vi "Tool Q LEIN High G Get buffer size.vi"(11 "error in (no error)":errorcluster) -> (15 "error out":errorcluster)   [LabVIEW 2011]
uses:
  LEINmaster/Defenitions/LEIN Structure variations.ctl
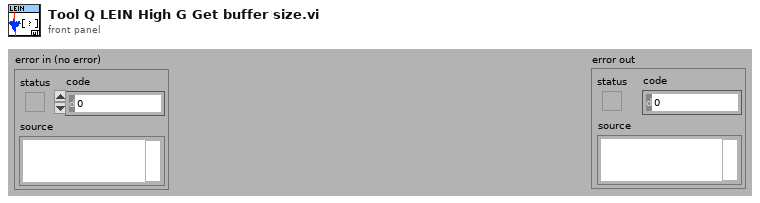
[diagram p1: front panel]
types:
  T1 = typedef "LEIN Structure variations.ctl" = enum16{"LEIN08", "LEIN31", "LEIN63"}
  T2 = typedef "LEIN CMD Cluster.ctl" = cluster{"SID":u8, "ANF":bool, "CMD":T3, "DATA":u8[]}
  T3 = typedef "LEIN CMD List.ctl" = enum8{"ACTI", "TASK", "RES0", "STAT", "RES1", "RES2", "RES3", "USER"}
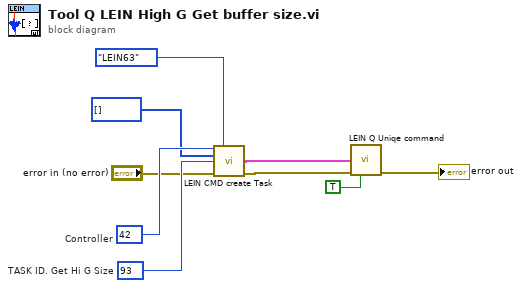
[diagram p0: block diagram]
diagram:
  w5 = u8 42  # Controller
  w7 = u8 93  # TASK ID. Get Hi G Size
  n1 = call "LEIN CMD create Task.vi"("SID"=w5, "LEIN Variation"=LEIN_Structure_variations."LEIN63", "Data"=u8[] [], "TASK ID"=w7, "error in (no error)"="error in (no error)") -> ("CMD"=w2:T2, "error out"=w4:errorcluster)  [unwired: 9 in]
  n2 = call "LEIN Q Uniqe command.vi"("CMD"=w2, "error in"=w4, "priority(F)"=TRUE) -> ("error out"=→"error out":errorcluster)  [unwired: 12 in]
